vi "Wait for PXI Interrupt Events.vi"(8 "error in (no error)":errorcluster, 10 "timeout ms (1000)":u32=1000, 11 "GE 5565PIORC in":refnum<class "GE 5565PIORC Old.lvclass">) -> (0 "error out":errorcluster, 2 "Timed out?":bool, 3 "GE 5565PIORC out":refnum<class "GE 5565PIORC Old.lvclass">)   [LabVIEW 2016, in "GE 5565PIORC Old.lvclass"]
uses:
  GE 5565PIORC Old.lvclass
  GE 5565PIORC Old.lvclass/GE 5565PIORC Old.ctl
  <vilib>/Instr/_visa.llb/Select Event Type.ctl
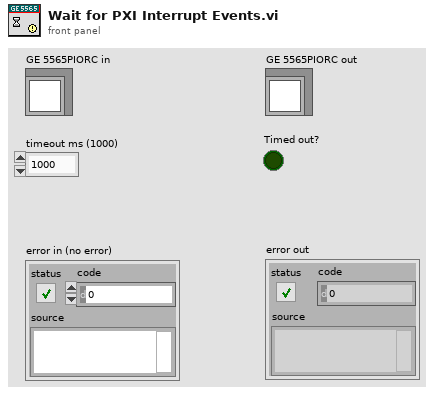
[diagram p1: front panel]
types:
  T1 = typedef "Select Event Type.ctl" = u32
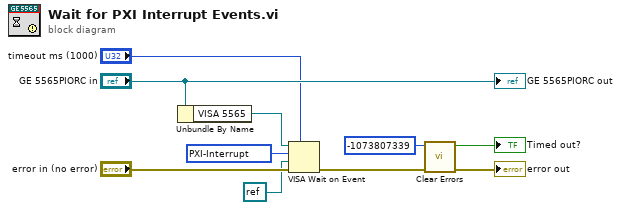
[diagram p0: block diagram]
diagram:
  w10 = T1 1073684514 items=["ServiceRequest"=1073684491, "Trigger"=3221168138, "Clear"=1073684493, "VXI-Signal"=1073684512, "VXI/VME-Interrupt"=3221168161, "VXI/VME-Sysfail"=1073684509, "VXI/VME-Sysreset"=1073684510, "GPIB-CIC"=1073684498, "GPIB-Talk"=1073684499, "GPIB-Listen"=1073684500, "PXI-Interrupt"=1073684514, "AllEnabled"=1073709055] ("Event Type")
  n1 = Unbundle By Name("GE 5565PIORC in") -> ("VISA 5565"=w8:refnum<visa-resource-name>)
  n2 = VISA Wait on Event(7:"timeout ms (1000)", 8:"error in (no error)", 9:refnum<visa-resource-name> refnum ("event class (Generic Event)"), 10:w10, 11:w8) -> (0:w3:errorcluster)  [unwired: 3 out]
  n3 = call <vilib>:"Clear Errors.vi"("error in (no error)"=w3, "specific error code to clear (0: all)"=-1073807339) -> ("error out"=→"error out":errorcluster, "specific error cleared?"=→"Timed out?":bool)  [unwired: 4 in]
  "GE 5565PIORC out" <- "GE 5565PIORC in"
